vi "Build Data Log Archive Path.vi"(0 "Log Directory String Array":string[](array[string])) -> (4 "Log Archive Directory String Array":string[](array[string]))   [LabVIEW 2027, in "Embedded Data Logger Scripting.lvlib"]
uses:
  Embedded Data Logger Scripting.lvlib
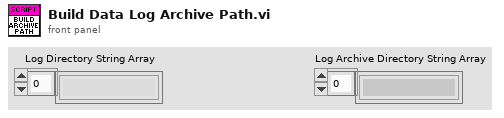
[diagram p1: front panel]
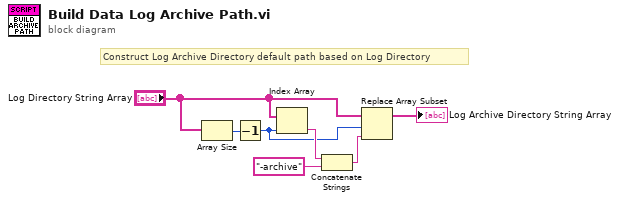
[diagram p0: block diagram]
diagram:
  # "Construct Log Archive Directory default path based on Log Directory"
  n1 = Array Size(array="Log Directory String Array") -> (size(s)=w1:i32)
  n2 = Decrement(x=w1) -> (x-1=w2:i32)
  n3 = Index Array(array="Log Directory String Array", index=w2) -> (element=w4:string)
  n4 = Concatenate Strings(w4, "-archive") -> (w5:string)
  n5 = Replace Array Subset(array="Log Directory String Array", new element=w5, index=w2) -> (→"Log Archive Directory String Array":string[])
